vi "Disable_Enable_Controls.vi"(0 "Disable_Control":refnum<vi>[](array[refnum]), 5 "Enable_Control":refnum<vi>[](array[refnum]), 11 "Error_In":errorcluster) -> (15 "Error_Out":errorcluster)   [LabVIEW 2021]
doc: "Used to disable and enable the controls."
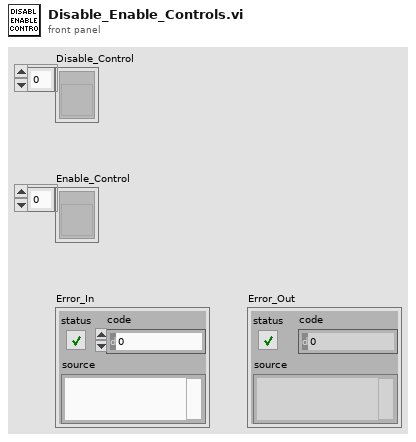
[diagram p1: front panel]
types:
  T1 = enum8{"Enabled", "Disabled", "Disabled and Grayed Out"}
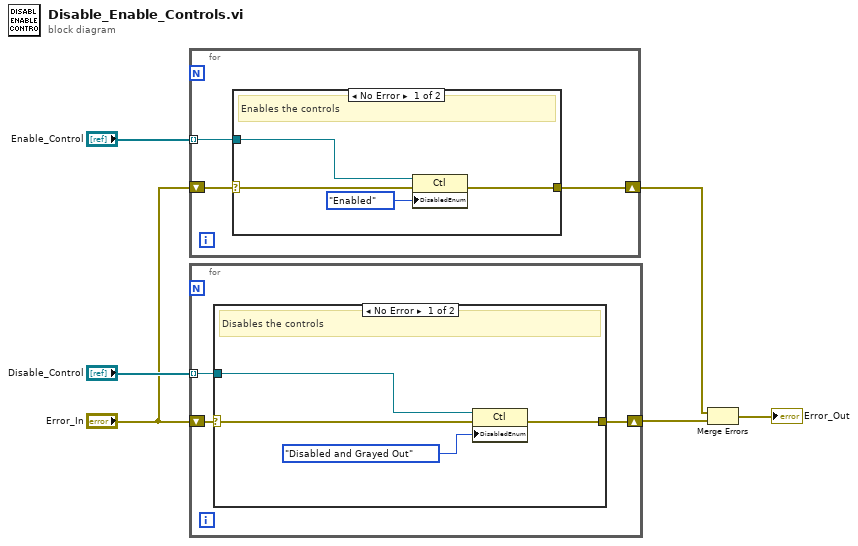
[diagram p0: block diagram]
diagram:
  n1 = for {
    shift-right: [w9] -> w1
    shift-left: "Error_In" -> [w7]
    tunnel: "Enable_Control" -> [w8] mode=indexing
    n2 = case shown="No Error" w7 {
      selector: w7 -> [w10 w14]
      tunnel: [w13 w14] -> w9
      tunnel: w8 -> [w12 _]
      frame No Error {
        # "Enables the controls"
        n3 = property class="Ctl"(reference=w12, error in=w10, "DisabledEnum"=T1."Enabled" ("Disabled")) -> (error out=w13:errorcluster)  [unwired: 1 out]
      }
      frame Error {
      }
    }
  }
  n4 = for {
    shift-right: [w17] -> w3
    shift-left: "Error_In" -> [w15]
    tunnel: "Disable_Control" -> [w16] mode=indexing
    n5 = case shown="No Error" w15 {
      selector: w15 -> [w18 w22]
      tunnel: [w21 w22] -> w17
      tunnel: w16 -> [w20 _]
      frame No Error {
        # "Disables the controls"
        n6 = property class="Ctl"(reference=w20, error in=w18, "DisabledEnum"=T1."Disabled and Grayed Out" ("Disabled")) -> (error out=w21:errorcluster)  [unwired: 1 out]
      }
      frame Error {
      }
    }
  }
  n7 = Merge Errors(w1, w3) -> (→"Error_Out":errorcluster)
